vi "读D32位.vi"(8 "error out":errorcluster, 10 "读取D地址":i32, 11 "VISA resource name out":refnum<visa-resource-name>) -> (0 "error IO":errorcluster, 2 "数值":i32, 3 "VISA resource name out 2":refnum<visa-resource-name>)   [LabVIEW 2018]
uses:
  <vilib>/Instr/_visa.llb/VISA Configure Serial Port (Instr).vi
panel:
  out "连接的字符串 2":string
  out "连接的字符串":string
  out "通讯延时":u32
  out "读取缓冲区":string
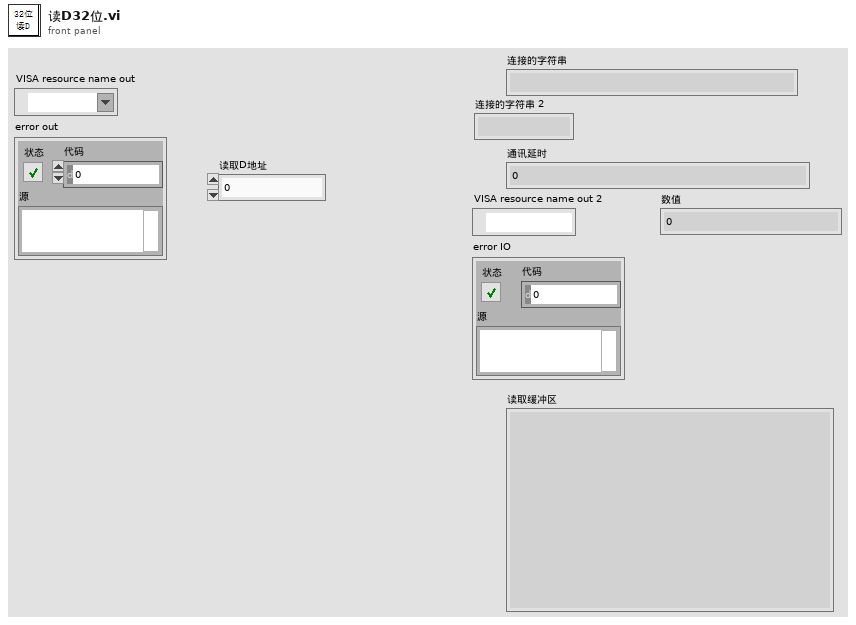
[diagram p1: front panel]
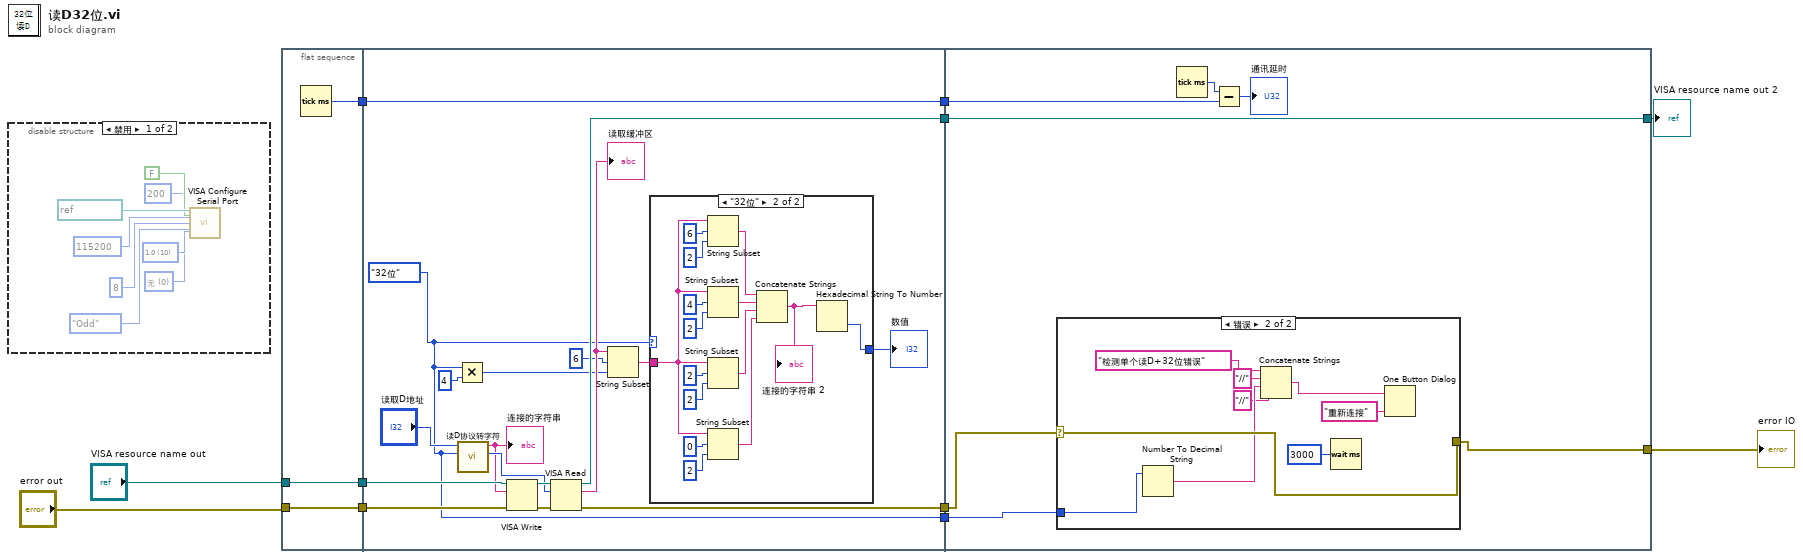
[diagram p0: block diagram]
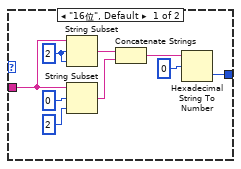
[diagram p3: hidden frame]
diagram:
  n1 = disable-structure shown="禁用" {
    frame Disabled {
      w13 = u16 0 items=["无", "XON/XOFF", "RTS/CTS", "XON/XOFF & RTS/CTS", "DTR/DSR", "XON/XOFF & DTR/DSR"] ("flow control (0:none)")
      w14 = u16 10 items=["1.0"=10, "1.5"=15, "2.0"=20] ("stop bits (10: 1 bit)")
      n2 = call-poly "VISA Configure Serial Port"("VISA resource name"=refnum<visa-resource-name> "COM3", "timeout (10sec)"=u32 200, "Enable Termination\nChar (T)"=FALSE ("Enable Termination\nChar (T)"), "baud rate (9600)"=u32 115200, "data bits (8)"=u16 8, "parity (0:none)"=enum16{"None", "Odd", "Even", "Mark", "Space"}."Odd", "stop bits (10: 1 bit)"=w14, "flow control (0:none)"=w13) -> ()  [unwired: 6 in, 2 out]
    }
    frame Enabled {
    }
  }
  n3 = flat-sequence {
    tunnel: [w22] -> w11
    tunnel: "VISA resource name out" -> [w21]
    tunnel: [w21] -> w10
    tunnel: [w20] -> w9
    tunnel: "error out" -> [w20]
    tunnel: w11 -> [w39]
    tunnel: [w39] -> w8
    tunnel: [w38] -> w7
    tunnel: [w37] -> w6
    tunnel: w10 -> [w36]
    tunnel: w9 -> [w35]
    tunnel: [w23] -> w1
    tunnel: w8 -> [w69]
    tunnel: w7 -> [w67]
    tunnel: [w67] -> w3
    tunnel: w6 -> [w66]
    tunnel: [w64] -> w2
    tunnel: w1 -> [w65]
    frame #0 {
      n4 = Tick Count (ms)() -> (millisecond timer value=w22:u32)
    }
    frame #1 {
      w23 = enum16{"默认", "16位", "32位"}."32位" ("枚举")
      n5 = Multiply(x=w23, y=4) -> (x*y=w28:i32)
      n6 = call "读D协议转字符.vi"("读取D个数"=w23, "读取D地址"="读取D地址") -> ("读取的字节数"=w32:i32, "连接的字符串"=w31:string)  [unwired: 8 in]
      "连接的字符串" <- w31
      n7 = VISA Write(VISA resource name=w36, write buffer=w31, error in (no error)=w35) -> (VISA resource name out=w34:refnum<visa-resource-name>, error out=w33:errorcluster)  [unwired: 1 out]
      n8 = VISA Read(VISA resource name=w34, byte count=w32, error in (no error)=w33) -> (VISA resource name out=w38:refnum<visa-resource-name>, read buffer=w30:string, error out=w37:errorcluster)  [unwired: 1 out]
      "读取缓冲区" <- w30
      n9 = String Subset(string=w30, offset (0)=6 ("偏移量(0)"), length (rest)=w28) -> (substring=w26:string)
      n10 = case shown="\"32位\"" w23 {
        tunnel: w26 -> [w46 w63]
        tunnel: [w40 w53] -> w25
        frame "16位", Default {
          w45 = 2 ("偏移量(0)")
          n11 = String Subset(string=w46, offset (0)=w45, length (rest)=w45) -> (substring=w43:string)
          n12 = String Subset(string=w46, offset (0)=0 ("偏移量(0)"), length (rest)=2 ("长度（剩余）")) -> (substring=w44:string)
          n13 = Concatenate Strings(w43, w44) -> (w42:string)
          n14 = Hexadecimal String To Number(string=w42, offset=0 ("偏移量")) -> (number=w40:u32)  [unwired: 1 in, 1 out]
        }
        frame "32位" {
          n15 = String Subset(string=w63, offset (0)=6 ("偏移量(0)"), length (rest)=2 ("长度（剩余）")) -> (substring=w58:string)
          n16 = String Subset(string=w63, offset (0)=4 ("偏移量(0)"), length (rest)=2 ("长度（剩余）")) -> (substring=w57:string)
          n17 = String Subset(string=w63, offset (0)=2 ("偏移量(0)"), length (rest)=2 ("长度（剩余）")) -> (substring=w56:string)
          n18 = String Subset(string=w63, offset (0)=0 ("偏移量(0)"), length (rest)=2 ("长度（剩余）")) -> (substring=w55:string)
          n19 = Concatenate Strings(w58, w57, w56, w55) -> (w54:string)
          "连接的字符串 2" <- w54
          n20 = Hexadecimal String To Number(string=w54) -> (number=w53:u32)  [unwired: 2 in, 1 out]
        }
      }
      "数值" <- w25
    }
    frame #2 {
      n21 = case shown="错误" w66 {
        selector: w66 -> [w71 w80]
        tunnel: [w71 w80] -> w64
        tunnel: w65 -> [_ w77]
        frame No Error {
        }
        frame Error {
          n22 = Number To Decimal String(number=w77) -> (decimal integer string=w74:string)  [unwired: 1 in]
          n23 = Concatenate Strings("检测单个读D+32位错误" ("消息"), "//" ("字符串"), w74, "//" ("字符串")) -> (w72:string)
          n24 = Wait (ms)(milliseconds to wait=u32 3000 ("等待时间（毫秒）")) -> ()  [unwired: 1 out]
          n25 = One Button Dialog(message=w72, button name ("OK")="重新连接" ("按钮名称（“确定”）")) -> ()  [unwired: 1 out]
        }
      }
      n26 = Tick Count (ms)() -> (millisecond timer value=w70:u32)
      n27 = Subtract(x=w70, y=w69) -> (x-y=→"通讯延时":u32)
    }
  }
  "VISA resource name out 2" <- w3
  "error IO" <- w2
